vi "new_subplot.vi"(9 "显示模式":i32, 10 "簇":T1, 11 "配置输入":T2 {"串口通信UI"."Format" items=["标准帧", "扩展帧"]; "串口通信UI"."Type" items=["数据帧", "远程帧"]; "串口通信UI"."ID" format="0x%x"; "串口通信UI"."Fliter" items=["接收所有类型"=1, "只接收标准帧"=2, "只接收扩展帧"=3]; "串口通信UI"."kBaudRate" items=["5k bps"=1, "10k bps"=2, "20k bps"=3, "40k bps"=4, "50k bps"=5, "80k bps"=6, "100k bps"=7, "125k bps"=8, "200k bps"=9, "250k bps"=10, "400k bps"=11, "500k bps"=12, "666k bps"=13, "800k bps"=14, "1000k bps"=15, "33.33k bps"=16, "66.66k bps"=17, "83.33k bps"=18]; "串口通信UI"."Mode" items=["正常工作", "仅侦听模式", "自测模式（环回）"]; "串口通信UI"."InitFlag" items=["使用界面设置参数"=1]; "串口通信UI"."AccMask" format="%08x"; "串口通信UI"."AccCode" format="%08x"; "串口通信UI"."Channel" items=["通道1", "通道2"]; "串口通信UI"."DevType" items=["USB-CAN"=3, "USB-CAN2"=4]; "安全报警UI"."操作 8" items=["产生报警信息（不发声），等待手动操作", "产生报警信息（发声），等待手动操作", "产生报警信息（不发声），自动刹车", "产生报警信息（发声），自动刹车", "产生报警信息（不发声），立即自动断电，开启泄放电阻", "产生报警信息（发声），立即自动断电，开启泄放电阻"]; "安全报警UI"."操作 7" items=["产生报警信息（不发声），等待手动操作", "产生报警信息（发声），等待手动操作", "产生报警信息（不发声），自动刹车", "产生报警信息（发声），自动刹车", "产生报警信息（不发声），立即自动断电，开启泄放电阻", "产生报警信息（发声），立即自动断电，开启泄放电阻"]; "安全报警UI"."操作 6" items=["产生报警信息（不发声），等待手动操作", "产生报警信息（发声），等待手动操作", "产生报警信息（不发声），自动刹车", "产生报警信息（发声），自动刹车", "产生报警信息（不发声），立即自动断电，开启泄放电阻", "产生报警信息（发声），立即自动断电，开启泄放电阻"]; "安全报警UI"."操作 5" items=["产生报警信息（不发声），等待手动操作", "产生报警信息（发声），等待手动操作", "产生报警信息（不发声），自动刹车", "产生报警信息（发声），自动刹车", "产生报警信息（不发声），立即自动断电，开启泄放电阻", "产生报警信息（发声），立即自动断电，开启泄放电阻"]; "安全报警UI"."操作 4" items=["产生报警信息（不发声），等待手动操作", "产生报警信息（发声），等待手动操作", "产生报警信息（不发声），自动刹车", "产生报警信息（发声），自动刹车", "产生报警信息（不发声），立即自动断电，开启泄放电阻", "产生报警信息（发声），立即自动断电，开启泄放电阻"]; "安全报警UI"."操作 3" items=["产生报警信息（不发声），等待手动操作", "产生报警信息（发声），等待手动操作", "产生报警信息（不发声），自动刹车", "产生报警信息（发声），自动刹车", "产生报警信息（不发声），立即自动断电，开启泄放电阻", "产生报警信息（发声），立即自动断电，开启泄放电阻"]; "安全报警UI"."操作 2" items=["产生报警信息（不发声），等待手动操作", "产生报警信息（发声），等待手动操作", "产生报警信息（不发声），自动刹车", "产生报警信息（发声），自动刹车", "产生报警信息（不发声），立即自动断电，开启泄放电阻", "产生报警信息（发声），立即自动断电，开启泄放电阻"]; "安全报警UI"."操作" items=["产生报警信息（不发声），等待手动操作", "产生报警信息（发声），等待手动操作", "产生报警信息（不发声），自动刹车", "产生报警信息（发声），自动刹车", "产生报警信息（不发声），立即自动断电，开启泄放电阻", "产生报警信息（发声），立即自动断电，开启泄放电阻"]}) -> (3 "配置输出":T2 {"串口通信UI"."Format" items=["标准帧", "扩展帧"]; "串口通信UI"."Type" items=["数据帧", "远程帧"]; "串口通信UI"."ID" format="0x%x"; "串口通信UI"."Fliter" items=["接收所有类型"=1, "只接收标准帧"=2, "只接收扩展帧"=3]; "串口通信UI"."kBaudRate" items=["5k bps"=1, "10k bps"=2, "20k bps"=3, "40k bps"=4, "50k bps"=5, "80k bps"=6, "100k bps"=7, "125k bps"=8, "200k bps"=9, "250k bps"=10, "400k bps"=11, "500k bps"=12, "666k bps"=13, "800k bps"=14, "1000k bps"=15, "33.33k bps"=16, "66.66k bps"=17, "83.33k bps"=18]; "串口通信UI"."Mode" items=["正常工作", "仅侦听模式", "自测模式（环回）"]; "串口通信UI"."InitFlag" items=["使用界面设置参数"=1]; "串口通信UI"."AccMask" format="%08x"; "串口通信UI"."AccCode" format="%08x"; "串口通信UI"."Channel" items=["通道1", "通道2"]; "串口通信UI"."DevType" items=["USB-CAN"=3, "USB-CAN2"=4]; "安全报警UI"."操作 8" items=["产生报警信息（不发声），等待手动操作", "产生报警信息（发声），等待手动操作", "产生报警信息（不发声），自动刹车", "产生报警信息（发声），自动刹车", "产生报警信息（不发声），立即自动断电，开启泄放电阻", "产生报警信息（发声），立即自动断电，开启泄放电阻"]; "安全报警UI"."操作 7" items=["产生报警信息（不发声），等待手动操作", "产生报警信息（发声），等待手动操作", "产生报警信息（不发声），自动刹车", "产生报警信息（发声），自动刹车", "产生报警信息（不发声），立即自动断电，开启泄放电阻", "产生报警信息（发声），立即自动断电，开启泄放电阻"]; "安全报警UI"."操作 6" items=["产生报警信息（不发声），等待手动操作", "产生报警信息（发声），等待手动操作", "产生报警信息（不发声），自动刹车", "产生报警信息（发声），自动刹车", "产生报警信息（不发声），立即自动断电，开启泄放电阻", "产生报警信息（发声），立即自动断电，开启泄放电阻"]; "安全报警UI"."操作 5" items=["产生报警信息（不发声），等待手动操作", "产生报警信息（发声），等待手动操作", "产生报警信息（不发声），自动刹车", "产生报警信息（发声），自动刹车", "产生报警信息（不发声），立即自动断电，开启泄放电阻", "产生报警信息（发声），立即自动断电，开启泄放电阻"]; "安全报警UI"."操作 4" items=["产生报警信息（不发声），等待手动操作", "产生报警信息（发声），等待手动操作", "产生报警信息（不发声），自动刹车", "产生报警信息（发声），自动刹车", "产生报警信息（不发声），立即自动断电，开启泄放电阻", "产生报警信息（发声），立即自动断电，开启泄放电阻"]; "安全报警UI"."操作 3" items=["产生报警信息（不发声），等待手动操作", "产生报警信息（发声），等待手动操作", "产生报警信息（不发声），自动刹车", "产生报警信息（发声），自动刹车", "产生报警信息（不发声），立即自动断电，开启泄放电阻", "产生报警信息（发声），立即自动断电，开启泄放电阻"]; "安全报警UI"."操作 2" items=["产生报警信息（不发声），等待手动操作", "产生报警信息（发声），等待手动操作", "产生报警信息（不发声），自动刹车", "产生报警信息（发声），自动刹车", "产生报警信息（不发声），立即自动断电，开启泄放电阻", "产生报警信息（发声），立即自动断电，开启泄放电阻"]; "安全报警UI"."操作" items=["产生报警信息（不发声），等待手动操作", "产生报警信息（发声），等待手动操作", "产生报警信息（不发声），自动刹车", "产生报警信息（发声），自动刹车", "产生报警信息（不发声），立即自动断电，开启泄放电阻", "产生报警信息（发声），立即自动断电，开启泄放电阻"]})   [LabVIEW 2018, in "UI.lvlib"]
uses:
  UI.lvlib
  Settings/Settings.ctl
  Acquisition/Hardware Configuration.ctl
  Acquisition/Signal Type.ctl
  Acquisition/Acquisition.lvlib
  Settings/Settings.lvlib
panel:
  # "参数配置文件"
  # "输入数据文件"
  # "EHA电机"
  # "模拟电机"
  # "注：每次运行实验时销毁现有所有图像"
  # "参数配置文件"
  # "输入数据文件"
  # "EHA电机"
  # "模拟电机"
  # "注：每次运行实验时销毁现有所有图像"
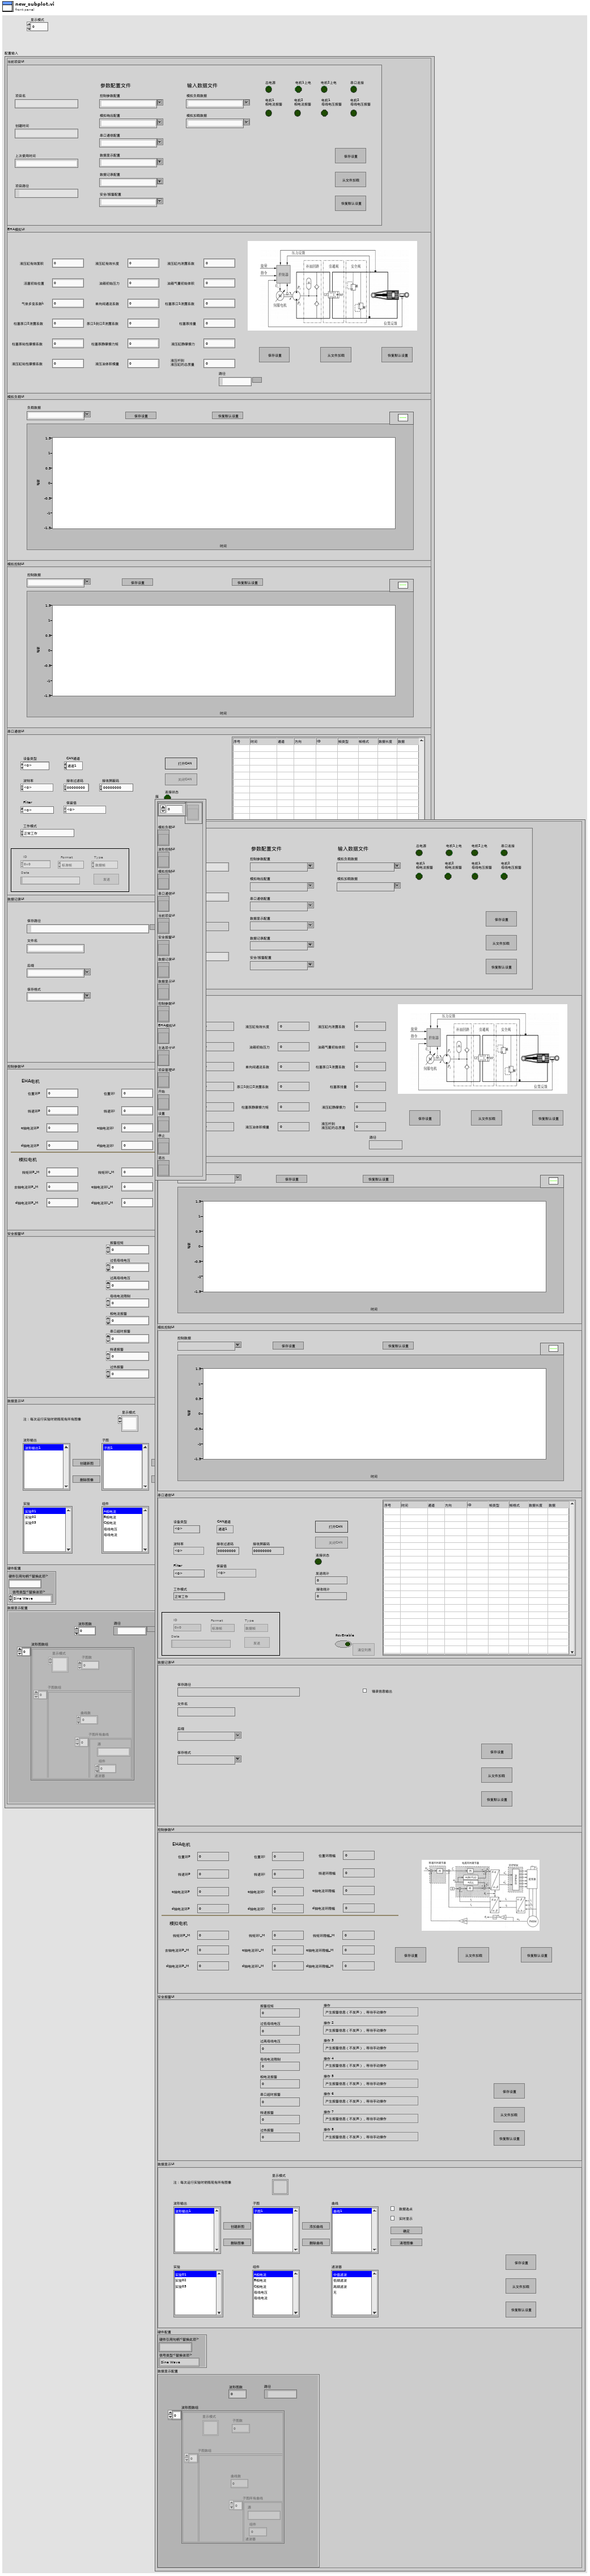
[diagram p1: front panel]
types:
  T1 = typedef "引用簇.ctl" = cluster{"数组":refnum<vi>[], "模拟负载UI":refnum<vi>, "波形控制UI":refnum<vi>, "模拟控制UI":refnum<vi>, "串口通信UI":refnum<vi>, "当前项目UI":refnum<vi>, "安全报警UI":refnum<vi>, "数据记录UI":refnum<vi>, "数据显示UI":refnum<vi>, "控制参数UI":refnum<vi>, "EHA模拟UI":refnum<vi>, "主选项卡UI":refnum<vi>, "项目管理UI":refnum<vi>, "开始":refnum<vi>, "设置":refnum<vi>, "停止":refnum<vi>, "退出":refnum<vi>}
  T2 = typedef "Settings.lvlib/Settings.ctl" = cluster{"当前项目UI":T3, "EHA模拟UI":T4, "模拟负载UI":T5, "模拟控制UI":T6, "串口通信UI":T7, "数据记录UI":T13, "控制参数UI":T14, "安全报警UI":T15, "数据显示UI":T16, "硬件配置":T17, "数据显示配置":T19}
  T3 = typedef "控件 5.ctl" = cluster{"控制参数配置":string, "模拟响应配置":string, "串口通信配置":string, "数据显示配置":string, "数据记录配置":string, "安全/报警配置":string, "模拟负载数据":string, "模拟加载数据":string, "总电源":bool, "电机1上电":bool, "电机2上电":bool, "串口连接":bool, "电机1\n相电流报警":bool, "电机2\n相电流报警":bool, "电机1\n母线电压报警":bool, "电机2\n母线电压报警":bool, "保存设置":bool, "从文件加载":bool, "恢复默认设置":bool, "路径":path, "项目路径":path, "项目名":string, "创建时间":string, "上次使用时间":string}
  T4 = typedef "EHA模拟UI.ctl" = cluster{"液压缸有效面积":dbl, "活塞初始位置":dbl, "气体多变系数k":dbl, "柱塞泵口2泄露系数":dbl, "柱塞泵粘性摩擦系数":dbl, "液压缸粘性摩擦系数":dbl, "液压缸有效长度":dbl, "油箱初始压力":dbl, "单向阀通流系数":dbl, "泵口1到口2泄露系数":dbl, "柱塞泵静摩擦力矩":dbl, "液压油体积模量":dbl, "保存设置":bool, "从文件加载":bool, "恢复默认设置":bool, "路径":path, "液压缸内泄露系数":dbl, "油箱气囊初始体积":dbl, "柱塞泵口1泄露系数":dbl, "柱塞泵排量":dbl, "液压缸静摩擦力":dbl, "液压杆到\n液压缸的总质量":dbl}
  T5 = typedef "控件 9.ctl" = cluster{"负载数据":string, "负载数据 2":waveform(dbl)[], "保存设置":bool, "恢复默认设置":bool}
  T6 = typedef "控件 7.ctl" = cluster{"控制数据":string, "负载数据 2":waveform(dbl)[], "保存设置":bool, "恢复默认设置":bool}
  T7 = typedef "控件 6.ctl" = cluster{"DevType":T8, "Channel":T9, "AccCode":u32, "AccMask":u32, "InitFlag":T10, "Mode":T11, "kBaudRate":u8, "Fliter":T12, "Open":bool, "Close":bool, "连接状态":bool, "SendCnt":u32, "RecvCnt":u32, "Send":bool, "ID":u32, "Data":string, "Type":u8, "Format":u8, "Clear":bool, "list":i32, "路径":path, "RcvEnable":bool}
  T8 = typedef "can库.lvlib/ControlCAN.lvlib/DevType.ctl" = u32
  T9 = typedef "can库.lvlib/ControlCAN.lvlib/CAN Channel.ctl" = u32
  T10 = typedef "can库.lvlib/ControlCAN.lvlib/InitFlag.ctl" = u32
  T11 = typedef "can库.lvlib/ControlCAN.lvlib/Mode.ctl" = u8
  T12 = typedef "can库.lvlib/ControlCAN.lvlib/Fliter.ctl" = u8
  T13 = typedef "控件 3.ctl" = cluster{"保存路径":path, "文件名":string, "后缀":string, "保存格式":string, "复选框":bool, "保存设置":bool, "从文件加载":bool, "恢复默认设置":bool, "路径":path, "TDMS文件引用":refnum<k34>}
  T14 = typedef "控件 1.ctl" = cluster{"d轴电流环P_M":dbl, "转速环P":dbl, "q轴电流环P":dbl, "d轴电流环P":dbl, "转矩环P_M":dbl, "去轴电流环P_M":dbl, "转速环I":dbl, "q轴电流环I":dbl, "d轴电流环I":dbl, "转矩环I_M":dbl, "q轴电流环I_M":dbl, "d轴电流环I_M":dbl, "保存设置":bool, "从文件加载":bool, "恢复默认设置":bool, "路径":path, "位置环P":dbl, "位置环I":dbl, "转速环限幅":dbl, "q轴电流环限幅":dbl, "d轴电流环限幅":dbl, "位置环限幅":dbl, "转矩环限幅_M":dbl, "q轴电流环限幅_M":dbl, "d轴电流环限幅_M":dbl}
  T15 = typedef "控件 4.ctl" = cluster{"报警扭矩":dbl, "过低母线电压":dbl, "过高母线电压":dbl, "母线电流限制":dbl, "相电流报警":dbl, "串口超时报警":dbl, "转速报警":dbl, "过热报警":dbl, "操作":u16, "操作 2":u16, "操作 3":u16, "操作 4":u16, "操作 5":u16, "操作 6":u16, "操作 7":u16, "操作 8":u16, "保存设置":bool, "从文件加载":bool, "恢复默认设置":bool, "路径":path}
  T16 = typedef "控件 2.ctl" = cluster{"保存设置":bool, "从文件加载":bool, "恢复默认设置":bool, "实验":i32, "波形输出":i32, "组件":i32, "曲线":i32, "滤波器":i32, "删除曲线":bool, "清理图像":bool, "添加曲线":bool, "数据选点":bool, "确定按钮":bool, "实时显示":bool, "子图":i32, "显示模式":u16, "路径":path, "删除图像":bool, "创建新图":bool}
  T17 = typedef "Acquisition.lvlib/Hardware Configuration.ctl" = cluster{"硬件引用句柄<替换此项>":string, "信号类型<替换该项>":T18}
  T18 = typedef "Acquisition.lvlib/Signal Type.ctl" = enum16{"Sine Wave", "Square with Noise"}
  T19 = typedef "波形图簇.ctl" = cluster{"波形图数":u32, "波形图数组":T20[], "路径":path}
  T20 = typedef "波形图.ctl" = cluster{"显示模式":u16, "子图数":u32, "子图数组":T21[]}
  T21 = typedef "子图.ctl" = cluster{"子图所有曲线":T22[], "曲线数":u32}
  T22 = typedef "曲线簇.ctl" = cluster{"源":string, "组件":u32, "滤波器":u32}
  T23 = enum8{"Enabled", "Disabled", "Disabled and Grayed Out"}
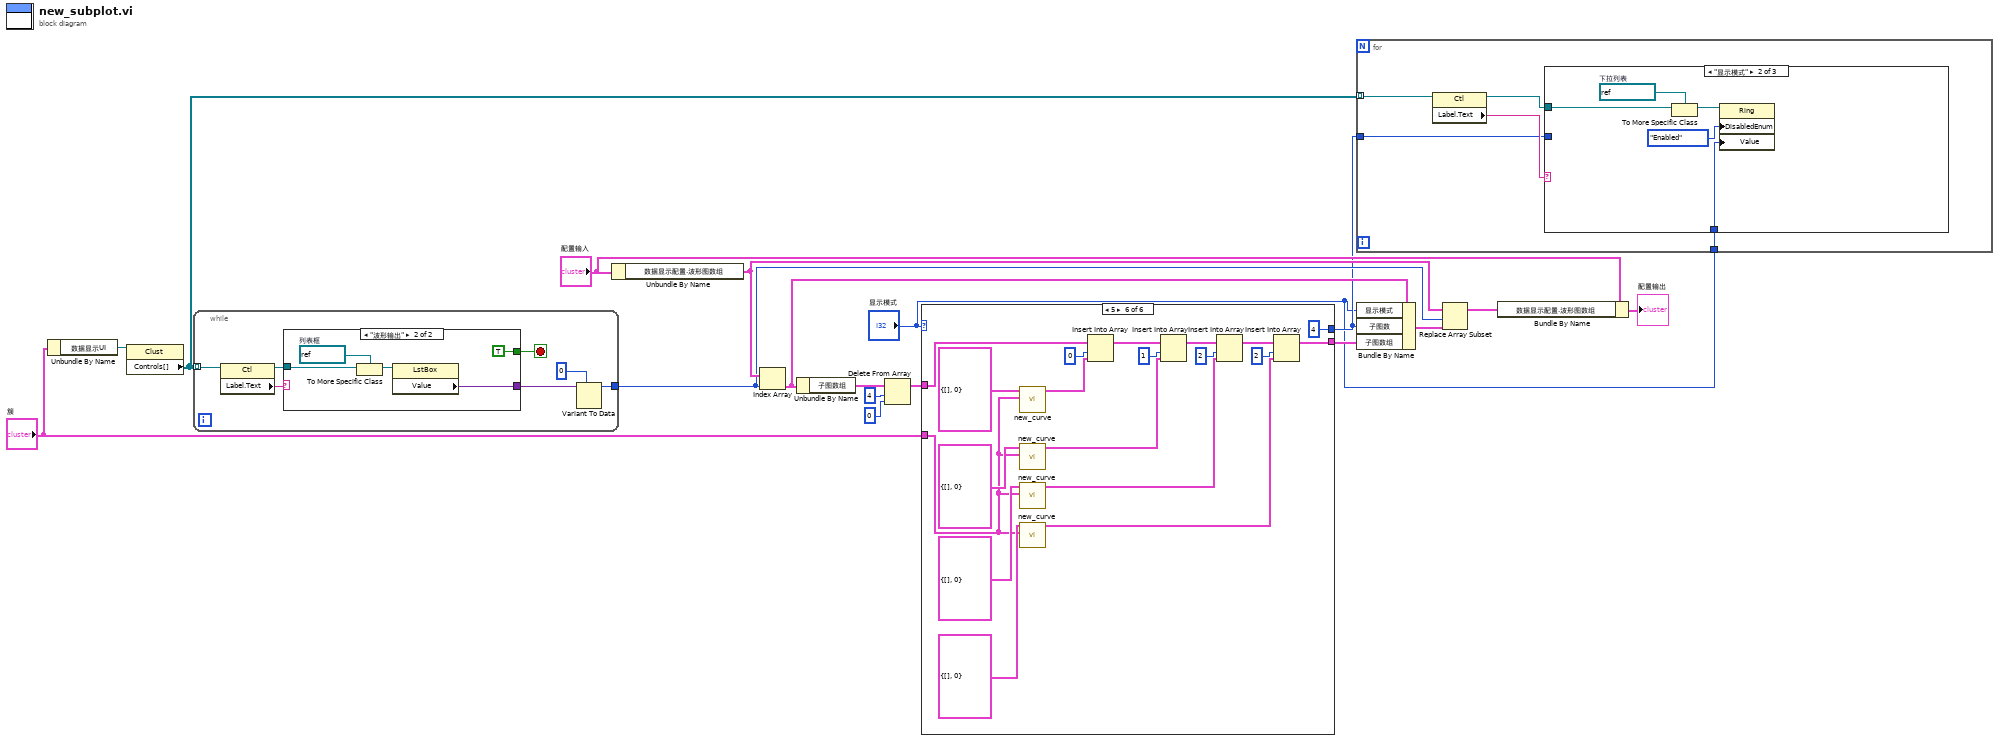
[diagram p0: block diagram]
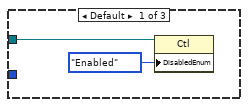
[diagram p2: hidden frame]
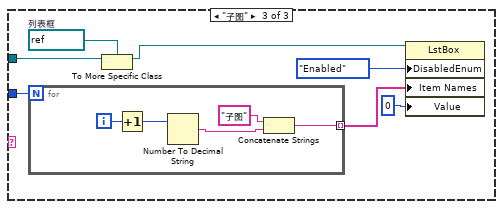
[diagram p3: hidden frame]
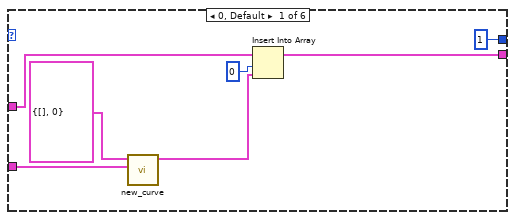
[diagram p4: hidden frame]
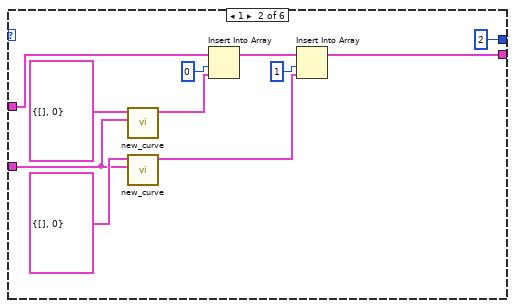
[diagram p5: hidden frame]
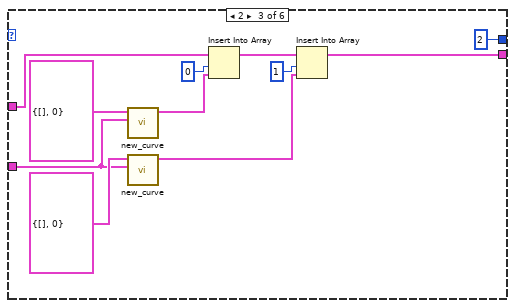
[diagram p6: hidden frame]
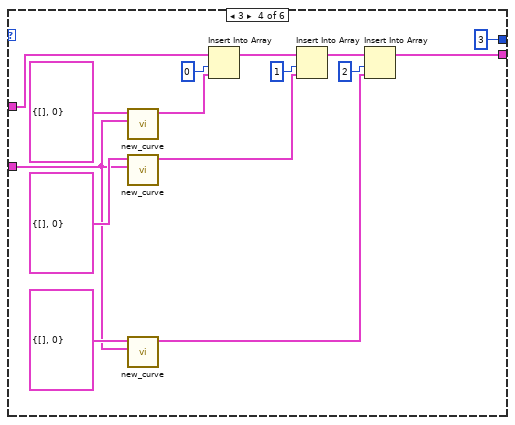
[diagram p7: hidden frame]
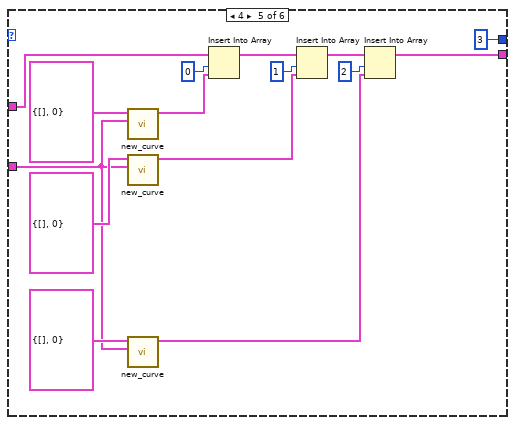
[diagram p8: hidden frame]
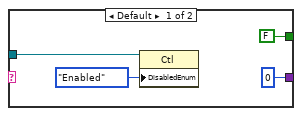
[diagram p9: hidden frame]
diagram:
  n1 = Unbundle By Name("簇") -> ("数据显示UI"=w17:refnum<vi>)
  n2 = property class="Clust"(reference=w17) -> ("Controls[]"=w6:refnum<vi>[])  [unwired: 1 in, 2 out]
  n3 = while {
    tunnel: w6 -> [w24] mode=indexing
    tunnel: [w19] -> w14
    stop <- w21 stop-if-true
    n4 = property class="Ctl"(reference=w24) -> (reference out=w22:refnum<vi>, "Label.Text"=w23:string)  [unwired: 1 in, 1 out]
    n5 = case shown="\"波形输出\"" w23 {
      tunnel: w22 -> [w28 w33]
      tunnel: [0 w29] -> w20
      tunnel: [FALSE TRUE] -> w21
      frame Default {
        n6 = property class="Ctl"(reference=w28, "DisabledEnum"=T23."Enabled" ("禁用")) -> ()  [unwired: 1 in, 2 out]
      }
      frame "波形输出" {
        w32 = refnum<vi> refnum  # 列表框
        n7 = To More Specific Class(target class=w32, reference=w33) -> (specific class reference=w31:refnum<vi>)  [unwired: 1 in, 1 out]
        n8 = property class="LstBox"(reference=w31) -> ("Value"=w29:variant)  [unwired: 1 in, 2 out]
      }
    }
    n9 = Variant To Data(type=0, Variant=w20) -> (data=w19:i32)  [unwired: 1 in, 1 out]
  }
  n10 = Unbundle By Name("配置输入") -> ("数据显示配置.波形图数组"=w15:T20[])
  n11 = Index Array(array=w15, index=w14) -> (element=w16:T20)
  n12 = Unbundle By Name(w16) -> ("子图数组"=w3:T21[])
  n13 = Delete From Array(array=w3, length=4 ("长度"), index=0 ("索引")) -> (array with subset deleted=w2:T21[])  [unwired: 1 out]
  n14 = case shown="5" "显示模式" {
    tunnel: [1 2 2 3 3 4] -> w7
    tunnel: "簇" -> [w39 w41 w52 w67 w82 w97]
    tunnel: w2 -> [w37 w49 w60 w75 w90 w109]
    tunnel: [w35 w42 w53 w64 w79 w93] -> w8
    frame 0, Default {
      n15 = call "new_curve.vi"("簇"=w39, "子图"=T21 {"子图所有曲线"=[], "曲线数"=0}) -> ("子图 2"=w36:T21)  [unwired: 9 in]
      n16 = Insert Into Array(array=w37, index=0 ("索引"), new element=w36) -> (w35:T21[])
    }
    frame 1 {
      n17 = call "new_curve.vi"("簇"=w41, "子图"=T21 {"子图所有曲线"=[], "曲线数"=0}) -> ("子图 2"=w48:T21)  [unwired: 9 in]
      n18 = call "new_curve.vi"("簇"=w41, "子图"=T21 {"子图所有曲线"=[], "曲线数"=0}) -> ("子图 2"=w45:T21)  [unwired: 9 in]
      n19 = Insert Into Array(array=w49, index=0 ("索引"), new element=w48) -> (w43:T21[])
      n20 = Insert Into Array(array=w43, index=1 ("索引"), new element=w45) -> (w42:T21[])
    }
    frame 2 {
      n21 = call "new_curve.vi"("簇"=w52, "子图"=T21 {"子图所有曲线"=[], "曲线数"=0}) -> ("子图 2"=w59:T21)  [unwired: 9 in]
      n22 = call "new_curve.vi"("簇"=w52, "子图"=T21 {"子图所有曲线"=[], "曲线数"=0}) -> ("子图 2"=w56:T21)  [unwired: 9 in]
      n23 = Insert Into Array(array=w60, index=0 ("索引"), new element=w59) -> (w54:T21[])
      n24 = Insert Into Array(array=w54, index=1 ("索引"), new element=w56) -> (w53:T21[])
    }
    frame 3 {
      n25 = call "new_curve.vi"("簇"=w67, "子图"=T21 {"子图所有曲线"=[], "曲线数"=0}) -> ("子图 2"=w74:T21)  [unwired: 9 in]
      n26 = call "new_curve.vi"("簇"=w67, "子图"=T21 {"子图所有曲线"=[], "曲线数"=0}) -> ("子图 2"=w71:T21)  [unwired: 9 in]
      n27 = call "new_curve.vi"("簇"=w67, "子图"=T21 {"子图所有曲线"=[], "曲线数"=0}) -> ("子图 2"=w63:T21)  [unwired: 9 in]
      n28 = Insert Into Array(array=w75, index=0 ("索引"), new element=w74) -> (w69:T21[])
      n29 = Insert Into Array(array=w69, index=1 ("索引"), new element=w71) -> (w65:T21[])
      n30 = Insert Into Array(array=w65, index=2 ("索引"), new element=w63) -> (w64:T21[])
    }
    frame 4 {
      n31 = call "new_curve.vi"("簇"=w82, "子图"=T21 {"子图所有曲线"=[], "曲线数"=0}) -> ("子图 2"=w89:T21)  [unwired: 9 in]
      n32 = call "new_curve.vi"("簇"=w82, "子图"=T21 {"子图所有曲线"=[], "曲线数"=0}) -> ("子图 2"=w86:T21)  [unwired: 9 in]
      n33 = call "new_curve.vi"("簇"=w82, "子图"=T21 {"子图所有曲线"=[], "曲线数"=0}) -> ("子图 2"=w78:T21)  [unwired: 9 in]
      n34 = Insert Into Array(array=w90, index=0 ("索引"), new element=w89) -> (w84:T21[])
      n35 = Insert Into Array(array=w84, index=1 ("索引"), new element=w86) -> (w80:T21[])
      n36 = Insert Into Array(array=w80, index=2 ("索引"), new element=w78) -> (w79:T21[])
    }
    frame 5 {
      n37 = call "new_curve.vi"("簇"=w97, "子图"=T21 {"子图所有曲线"=[], "曲线数"=0}) -> ("子图 2"=w108:T21)  [unwired: 9 in]
      n38 = call "new_curve.vi"("簇"=w97, "子图"=T21 {"子图所有曲线"=[], "曲线数"=0}) -> ("子图 2"=w105:T21)  [unwired: 9 in]
      n39 = call "new_curve.vi"("簇"=w97, "子图"=T21 {"子图所有曲线"=[], "曲线数"=0}) -> ("子图 2"=w99:T21)  [unwired: 9 in]
      n40 = call "new_curve.vi"("簇"=w97, "子图"=T21 {"子图所有曲线"=[], "曲线数"=0}) -> ("子图 2"=w95:T21)  [unwired: 9 in]
      n41 = Insert Into Array(array=w109, index=0 ("索引"), new element=w108) -> (w103:T21[])
      n42 = Insert Into Array(array=w103, index=1 ("索引"), new element=w105) -> (w100:T21[])
      n43 = Insert Into Array(array=w100, index=2 ("索引"), new element=w99) -> (w94:T21[])
      n44 = Insert Into Array(array=w94, index=2 ("索引"), new element=w95) -> (w93:T21[])
    }
  }
  n45 = for {
    tunnel: w7 -> [w113]
    tunnel: w6 -> [w116] mode=indexing
    tunnel: "显示模式" -> [w112]
    n46 = property class="Ctl"(reference=w116) -> (reference out=w115:refnum<vi>, "Label.Text"=w114:string)  [unwired: 1 in, 1 out]
    n47 = case shown="\"显示模式\"" w114 {
      tunnel: w115 -> [w118 w121 w125]
      tunnel: w113 -> [_ _ w124]
      tunnel: w112 -> [_ w119 _]
      frame Default {
        n48 = property class="Ctl"(reference=w118, "DisabledEnum"=T23."Enabled" ("禁用")) -> ()  [unwired: 1 in, 2 out]
      }
      frame "显示模式" {
        w122 = refnum<vi> refnum  # 下拉列表
        n49 = To More Specific Class(target class=w122, reference=w121) -> (specific class reference=w120:refnum<vi>)  [unwired: 1 in, 1 out]
        n50 = property class="Ring"(reference=w120, "DisabledEnum"=T23."Enabled" ("禁用"), "Value"=w119) -> ()  [unwired: 1 in, 2 out]
      }
      frame "子图" {
        w129 = refnum<vi> refnum  # 列表框
        n51 = for {
          N: w124 -> [_]
          tunnel: [w133] -> w127 mode=indexing
          i -> [w135]
          n52 = Increment(x=w135) -> (x+1=w131:i32)
          n53 = Number To Decimal String(number=w131) -> (decimal integer string=w132:string)  [unwired: 1 in]
          n54 = Concatenate Strings("子图", w132) -> (w133:string)
        }
        n55 = To More Specific Class(target class=w129, reference=w125) -> (specific class reference=w128:refnum<vi>)  [unwired: 1 in, 1 out]
        n56 = property class="LstBox"(reference=w128, "DisabledEnum"=T23."Enabled" ("禁用"), "Item Names"=w127, "Value"=0) -> ()  [unwired: 1 in, 2 out]
      }
    }
  }
  n57 = Bundle By Name(cluster=w16, "显示模式"="显示模式", "子图数"=w7, "子图数组"=w8) -> (w13:T20)
  n58 = Replace Array Subset(array=w15, new element=w13, index=w14) -> (w11:T20[])
  n59 = Bundle By Name(cluster="配置输入", "数据显示配置.波形图数组"=w11) -> (→"配置输出":T2)
